vi "Perform Measurement.vi"(7 "error in":errorcluster, 8 "Measure Call Context in":refnum<class "Measure Call Context.lvclass">, 10 "measurement configuration":T2={"Mode of operation"=enum."Power on the DUT", "Source resource names"=[], "Load resource names"=[], "Power ON output function"=1006, "Power ON/Source system configuration"=enum."Parallel", "Power ON V/I Source start level"=6.0, "Source stop voltage"=14.0, "Source voltage sweep points"=4, "Source voltage level range"=20.0, "Power ON/Source sense"=1009, "Source limit symmetry"=enum."Asymmetric", "Power ON/Source current/voltage limit range"=25.0, "Source current limit low"=-0.6, "Source current limit high"=25.0, "Source transient response"=1038, "Source voltage gain bandwidth"=2000.0, "Source voltage compensation frequency"=3530.0, "Source voltage pole-zero ratio"=2.0, "Load system configuration"=enum."Parallel", "Load device voltage/current rating"=50.0, "Load start current"=1.0, "Load stop current"=50.0, "Load current sweep points/points per decade"=10, "Load sweep type"="Logarithmic", "Load current level range"=80.0, "Load sense"=1009, "Load limit symmetry"=enum."Symmetric", "Load voltage limit range"=6.0, "Load voltage limit low"=0.0, "Load voltage limit high"=inf, "Load transient response"=1038, "Load current gain bandwidth"=14000.0, "Load current compensation frequency"=180000.0, "Load current pole-zero ratio"=0.3, "DUT setup time"=1.0, "Source delay"=0.005, "Aperture time"=0.005, "Nominal output voltage"=1.0, "Measurement timeout"=10.0} {"Power ON output function" items=["Series", "Parallel", "Manual"]; "Nominal output voltage" format="%#_6pA"; "Source stop voltage" format="%#_6p"; "Load stop current" format="%#_6p"; "Source voltage sweep points" format="%#_6p"; "Load sense" items=["Symmetric", "Asymmetric"]; "Load transient response" items=["Slow"=1041, "Normal"=1038, "Fast"=1039, "Custom"=1042]; "Power ON/Source sense" items=["Symmetric", "Asymmetric"]; "Source transient response" items=["Slow"=1041, "Normal"=1038, "Fast"=1039, "Custom"=1042]; "Load voltage limit high" format="%#_6p"; "Load voltage limit range" format="%#_6p"; "Load current level range" format="%#_6p"; "Source current limit high" format="%#_6p"; "Source current limit low" format="%#_6p"; "Power ON/Source current/voltage limit range" format="%#_6p"; "Source voltage level range" format="%#_6p"}) -> (0 "error out":errorcluster, 1 "Measure Call Context out":refnum<class "Measure Call Context.lvclass">, 3 "measurement results":T1)   [LabVIEW 2021, in "Eff And Load Reg_Channel Ganging.lvlib"]
doc: "Perform the calling of API in proper sequence to take Efficency and Load regulation measurement in different configurations of source and load like\n\nSingle-Single\nSingle-Ganged\nGanged-Single\nGanged-Ganged"
uses:
  Eff And Load Reg_Channel Ganging.lvlib
  shared subVIs/ctl/NIDCPower_channel_ganging - ctl - ganged config.ctl
  shared subVIs/ctl/NIDCPower_channel_ganging - ctl - channel mode.ctl
  shared/Single/controls/Initialize Resource Config-Single.ctl
  shared/Ganging/controls/Initialize Resource Config-Ganging.ctl
  shared subVIs/ctl/NIDCPower_channel_ganging - ctl - ganged session.ctl
  <instrlib>/niDCPower/nidcpower.llb/niDCPower Wait For Event - Event.ctl
  shared/Single/controls/Source to Sequence Config-Single.ctl
  shared/Ganging/controls/Source to Sequence Config-Ganging.ctl
  shared/Single/controls/Load to Sequence Config-Single.ctl
  shared/Ganging/controls/Load to Sequence Config-Ganging.ctl
  shared/Common/controls/Start and Wait for Event.ctl
  shared/Ganging/controls/Abort Single Point-Ganging.ctl
  shared/Single/controls/Abort Single Point-Single.ctl
  <instrlib>/niDCPower/nidcpower.llb/niDCPower Output Function.ctl
  Measurement Results.ctl
  Controls/Efficency perform meaasurement.ctl
  Controls/Efficency fetch measurement control.ctl
  <vilib>/Plug-In SDKs/Measurements/Measure Call Context/Measure Call Context.lvclass
  Measurement Configuration.ctl
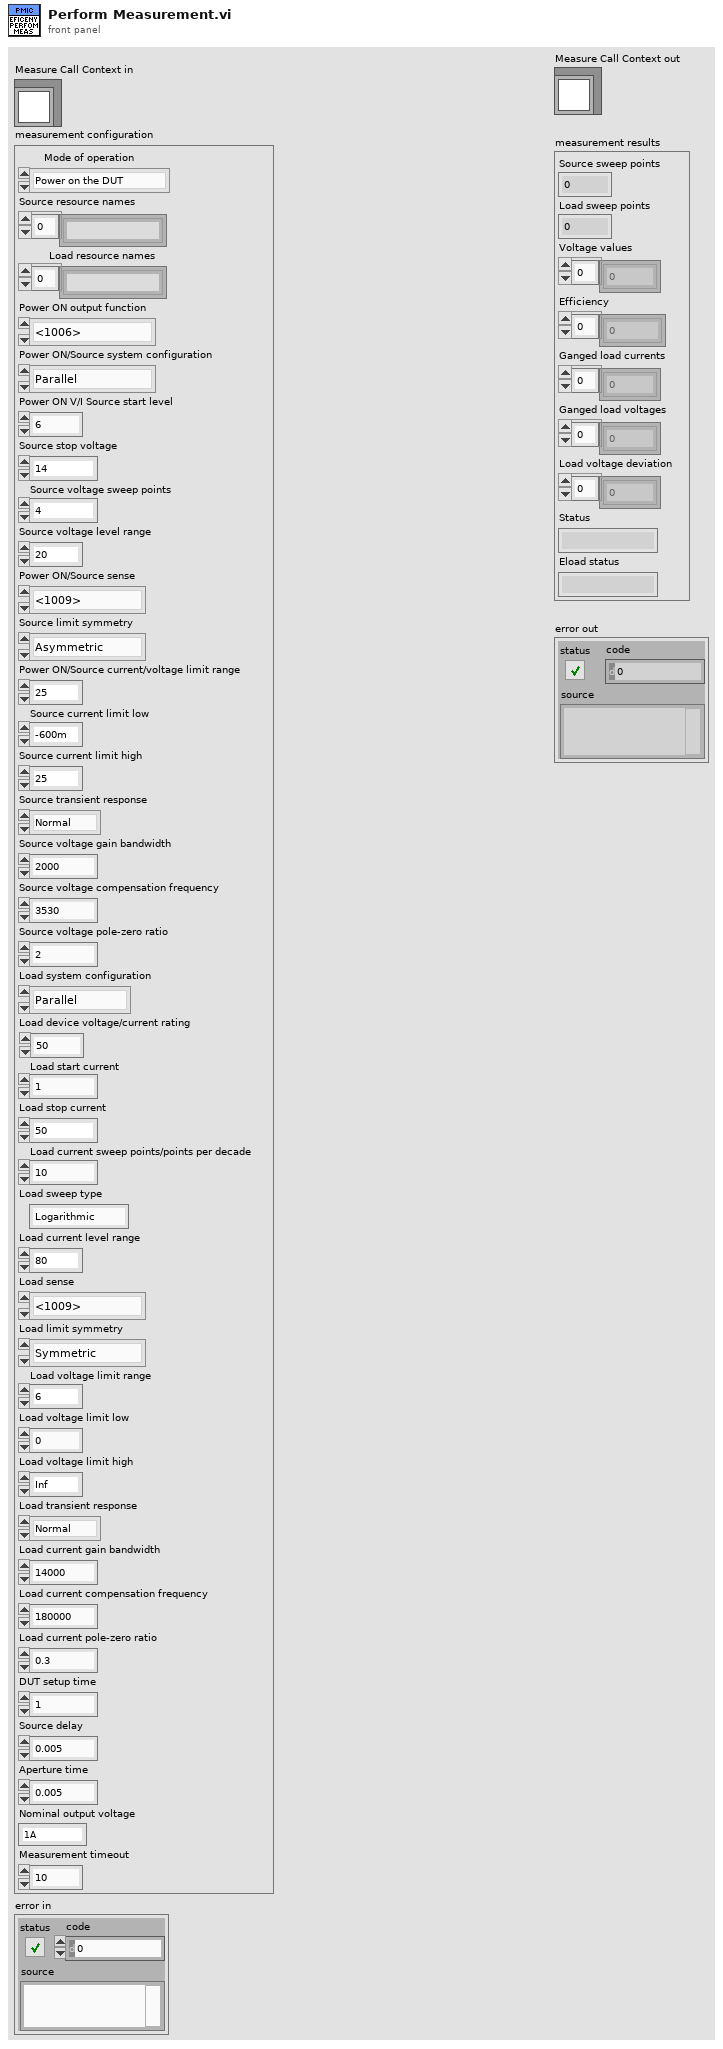
[diagram p1: front panel]
types:
  T1 = typedef "Eff And Load Reg_Channel Ganging.lvlib/Measurement Results.ctl" = cluster{"Source sweep points":i32, "Load sweep points":i32, "Voltage values":dbl[], "Efficiency":dbl[], "Ganged load currents":dbl[], "Ganged load voltages":dbl[], "Load voltage deviation":dbl[], "Status":string, "Eload status":string}
  T2 = typedef "Eff And Load Reg_Channel Ganging.lvlib/Measurement Configuration.ctl" = cluster{"Mode of operation":enum32{"Power on the DUT", "Perform measurement", "Power off the DUT"}, "Source resource names":string[], "Load resource names":string[], "Power ON output function":i32, "Power ON/Source system configuration":enum32{"Series", "Parallel", "Manual"}, "Power ON V/I Source start level":dbl, "Source stop voltage":dbl, "Source voltage sweep points":i32, "Source voltage level range":dbl, "Power ON/Source sense":i32, "Source limit symmetry":enum32{"Symmetric", "Asymmetric"}, "Power ON/Source current/voltage limit range":dbl, "Source current limit low":dbl, "Source current limit high":dbl, "Source transient response":i32, "Source voltage gain bandwidth":dbl, "Source voltage compensation frequency":dbl, "Source voltage pole-zero ratio":dbl, "Load system configuration":enum32{"Series", "Parallel", "Manual"}, "Load device voltage/current rating":dbl, "Load start current":dbl, "Load stop current":dbl, "Load current sweep points/points per decade":i32, "Load sweep type":string, "Load current level range":dbl, "Load sense":i32, "Load limit symmetry":enum32{"Symmetric", "Asymmetric"}, "Load voltage limit range":dbl, "Load voltage limit low":dbl, "Load voltage limit high":dbl, "Load transient response":i32, "Load current gain bandwidth":dbl, "Load current compensation frequency":dbl, "Load current pole-zero ratio":dbl, "DUT setup time":dbl, "Source delay":dbl, "Aperture time":dbl, "Nominal output voltage":dbl, "Measurement timeout":dbl}
  T3 = typedef "Eff And Load Reg_Channel Ganging.lvlib/Efficency perform meaasurement.ctl" = cluster{"Source Ganged Session Out":T4, "Load Ganged Session Out":T4, "Source sweep values":dbl[], "Source sweep points":i32, "Load sweep values":dbl[], "Load sweep points":i32, "Source Master/Single resource name":string, "Source Slave resource name":string[], "Load Master/Single resource name":string, "Load Slave resource name":string[], "Load ganged/single":bool, "Source ganged/single":bool, "Source trigger":string, "measure trigger":string, "Source channel name":string, "Load channel name":string, "Source session out":refnum<k15>, "Load session out":refnum<k15>, "measurement results":T1, "Number of Eload used":i32}
  T4 = typedef "NIDCPower_channel_ganging - ctl - ganged session.ctl" = cluster{"Ganged Config":T5, "Session List":refnum<k15>[], "Session Mode":T6[], "Channel":string[]}
  T5 = typedef "NIDCPower_channel_ganging - ctl - ganged config.ctl" = enum32{"Series", "Parallel", "Manual"}
  T6 = typedef "NIDCPower_channel_ganging - ctl - channel mode.ctl" = enum32{"Master", "Slave", "Slave - Inverted"}
  T7 = typedef "Initialize Resource Config-Single.ctl" = cluster{"Resource name":string, "Voltage/current level":dbl, "Voltage/current level range":dbl, "Voltage/current limit range":dbl, "Voltage/current limit low":dbl, "Voltage/current limit high":dbl, "Output function":i32, "Sense":i32, "Transient response":i32, "Voltage/current gain bandwidth":dbl, "Voltage/current compensation frequency":dbl, "Voltage/current pole-zero ratio":dbl, "DUT set-up time":dbl, "Limit symmetry":enum32{"Symmetric", "Asymmetric"}}
  T8 = typedef "Initialize Resource Config-Ganging.ctl" = cluster{"Master resource name ":string, "Slave resource names":string[], "System configuration":enum32{"Series", "Parallel", "Manual"}, "Voltage/current level":dbl, "Voltage/current level range":dbl, "Limit symmetry":enum32{"Symmetric", "Asymmetric"}, "Voltage/current limit range":dbl, "Voltage/current limit low":dbl, "Voltage/current limit high":dbl, "Output function":i32, "Sense":i32, "Transient response":i32, "Voltage/current gain bandwith":dbl, "Voltage/current compensation frequency":dbl, "Voltage/current pole-zero ratio":dbl, "DUT set-up time":dbl}
  T9 = typedef "Source to Sequence Config-Single.ctl" = cluster{"Source channel name":string, "Source out":refnum<k15>, "Source sweep values":dbl[], "Load sweep points":i32, "Source output function":i32, "Source transient response":i32, "Source voltage/current gain bandwidth":dbl, "Source voltage/current compensation frequency":dbl, "Source voltage/current pole-zero ratio":dbl, "Source aperture time":dbl, "Source source delay":dbl}
  T10 = typedef "Source to Sequence Config-Ganging.ctl" = cluster{"Source Ganged Session Out":cluster{"Ganged Config":T5, "Session List":refnum<k15>[], "Session Mode":T6[], "Channel":string[]}, "Source sweep values":dbl[], "Load sweep points":i32, "Source output function":i32, "Source transient response":i32, "Source voltage/current gain bandwidth":dbl, "Source voltage/current compensation frequency":dbl, "Source voltage/current pole-zero ratio":dbl, "Source aperture time":dbl, "Source source delay":dbl}
  T11 = typedef "Load to Sequence Config-Single.ctl" = cluster{"Load channel name":string, "Load out":refnum<k15>, "Load sweep values":dbl[], "Source sweep points":i32, "Load output function":i32, "Load transient response":i32, "Load voltage/current gain bandwidth":dbl, "Load voltage/current compensation frequency":dbl, "Load voltage/current pole-zero ratio":dbl, "Load aperture time":dbl, "Load source delay":dbl, "Load measure trigger":string, "Load source trigger":string}
  T12 = typedef "Load to Sequence Config-Ganging.ctl" = cluster{"Load Ganged Session Out":cluster{"Ganged Config":T5, "Session List":refnum<k15>[], "Session Mode":T6[], "Channel":string[]}, "Load sweep values":dbl[], "Source sweep points":i32, "Load output function":i32, "Load transient response":i32, "Load voltage/current gain bandwidth":dbl, "Load voltage/current compensation frequency":dbl, "Load voltage/current pole-zero ratio":dbl, "Load aperture time":dbl, "Load source delay":dbl, "Load measure trigger":string, "Load source trigger":string}
  T13 = enum16{"SOURCE AND LOAD OFF", "SOURCE ON", "LOAD ON", "SOURCE AND LOAD ON"}
  T14 = typedef "Start and Wait for Event.ctl" = cluster{"Source Ganged Session Out":T4, "Load Ganged Session Out":T4, "Source session out":refnum<k15>, "Load session out":refnum<k15>, "event":T15, "Source channel name":string, "Load channel name":string, "Load Source ON/OFF":enum16{"SOURCE AND LOAD OFF", "SOURCE ON", "LOAD ON", "SOURCE AND LOAD ON"}, "Load ganged/single":bool, "Source ganged/single":bool}
  T15 = typedef "niDCPower Wait For Event - Event.ctl" = i32
  T16 = typedef "Eff And Load Reg_Channel Ganging.lvlib/Efficency fetch measurement control.ctl" = cluster{"Load,Source ON&OFF":u32, "Source Ganged Session Out":T4, "Load Ganged Session Out":T4, "Source sweep values":dbl[], "Source sweep points":i32, "Load sweep values":dbl[], "Load sweep points":i32, "Load ganged/single":bool, "Source ganged/single":bool, "Source channel name":string, "Load channel name":string, "Source session out":refnum<k15>, "Load session out":refnum<k15>, "measurement results":T1, "Nominal output voltage":dbl, "Measurement timeout":dbl}
  T17 = typedef "Abort Single Point-Ganging.ctl" = cluster{"Ganged Session in":cluster{"Ganged Config":T5, "Session List":refnum<k15>[], "Session Mode":T6[], "Channel":string[]}}
  T18 = typedef "Abort Single Point-Single.ctl" = cluster{"Resource out":refnum<k15>, "Resource channel name":string}
  T19 = enum32{"Power on the DUT", "Perform measurement", "Power off the DUT"}
  T20 = typedef "niDCPower Output Function.ctl" = i32
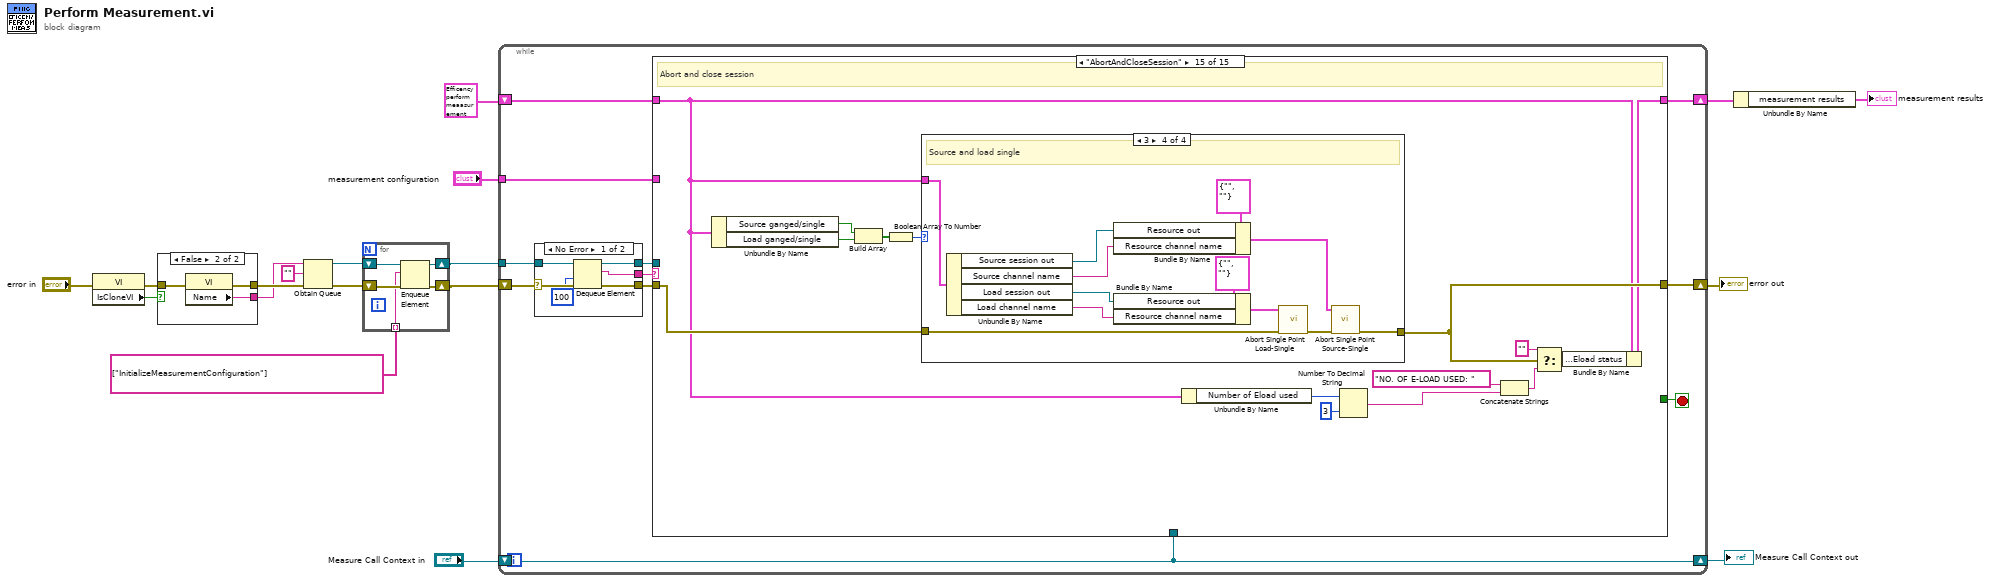
[diagram p0: block diagram]
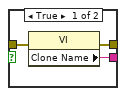
[diagram p2: hidden frame]
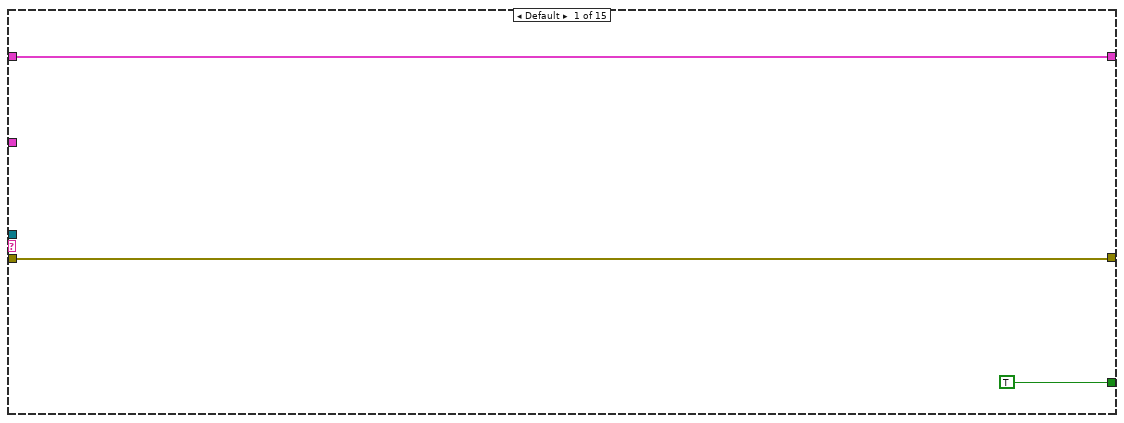
[diagram p3: hidden frame]
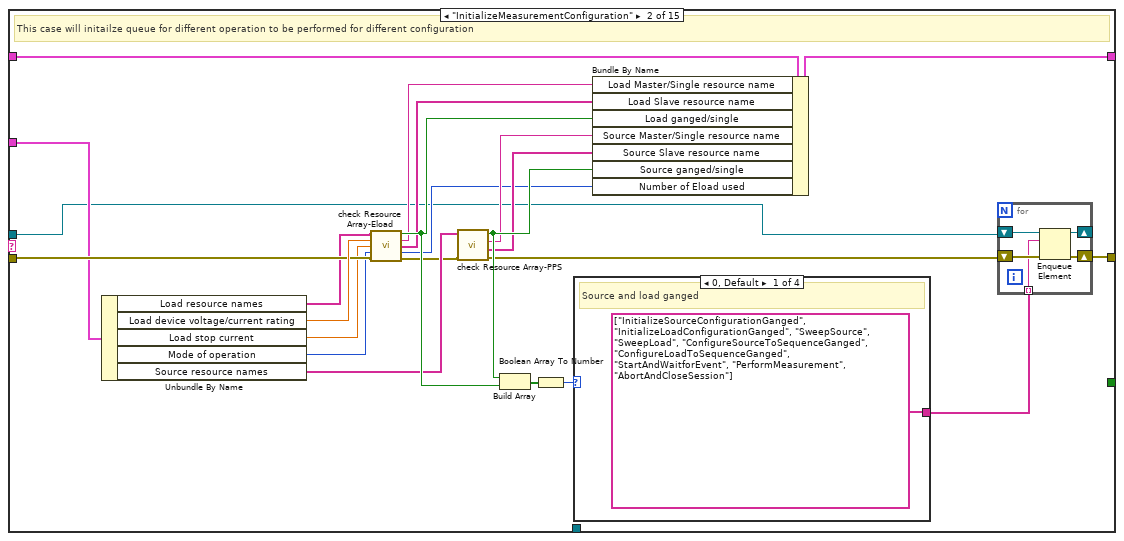
[diagram p4: hidden frame]
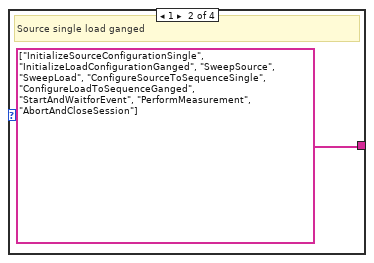
[diagram p5: hidden frame]
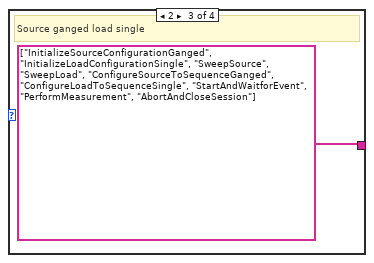
[diagram p6: hidden frame]
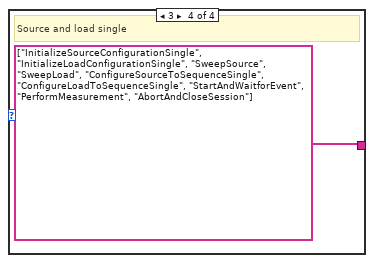
[diagram p7: hidden frame]
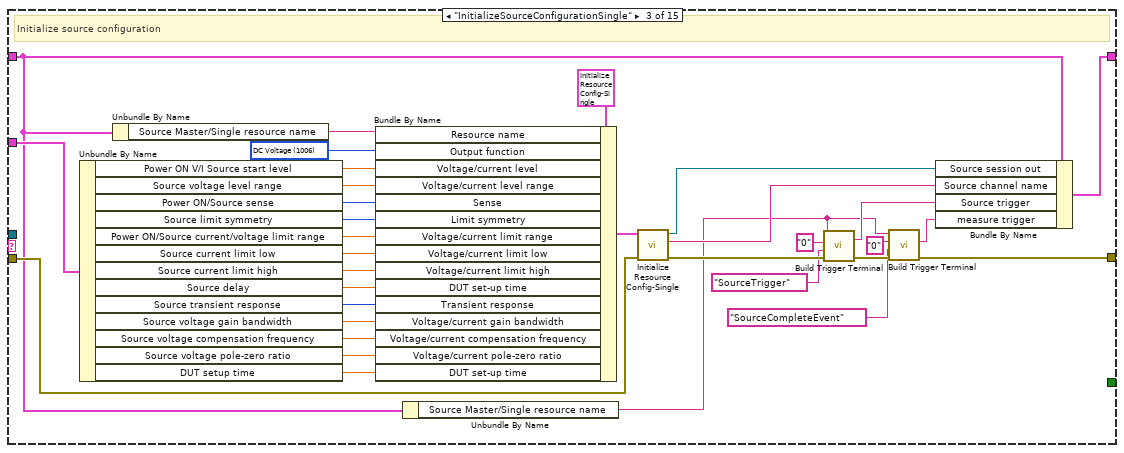
[diagram p8: hidden frame]
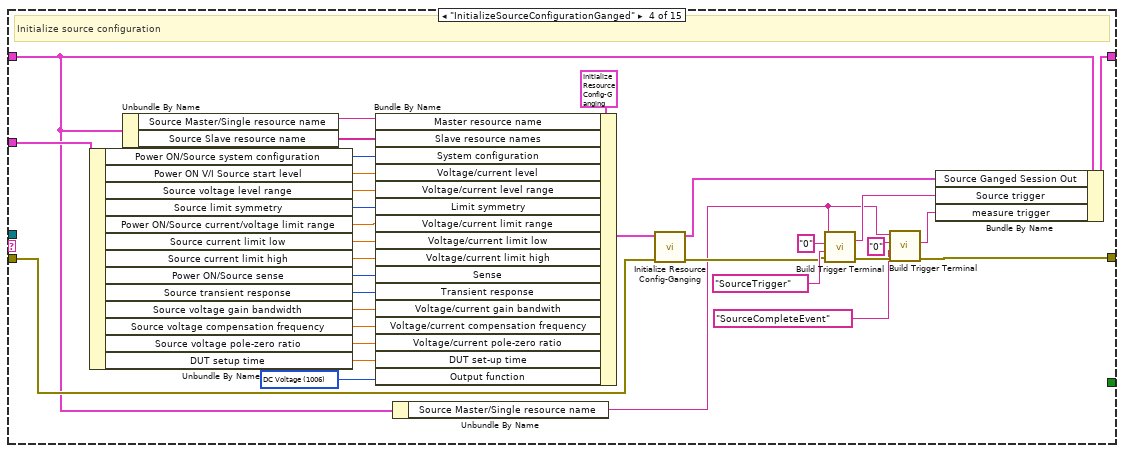
[diagram p9: hidden frame]
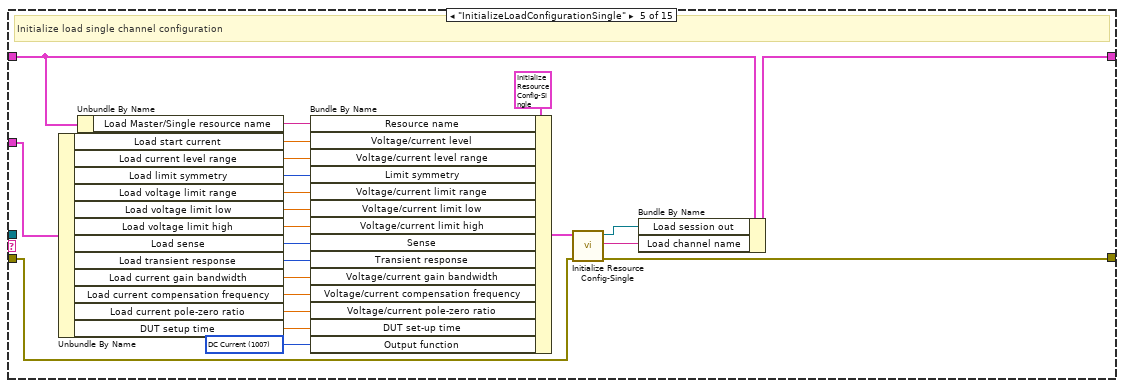
[diagram p10: hidden frame]
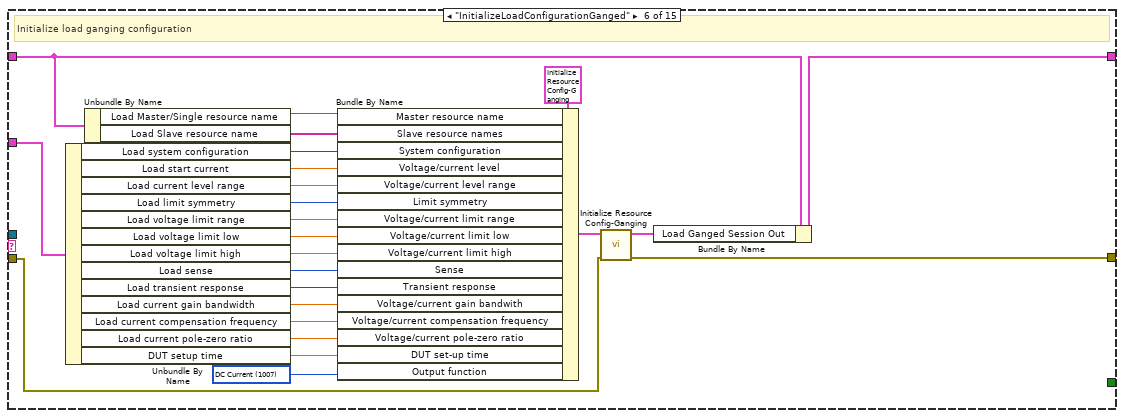
[diagram p11: hidden frame]
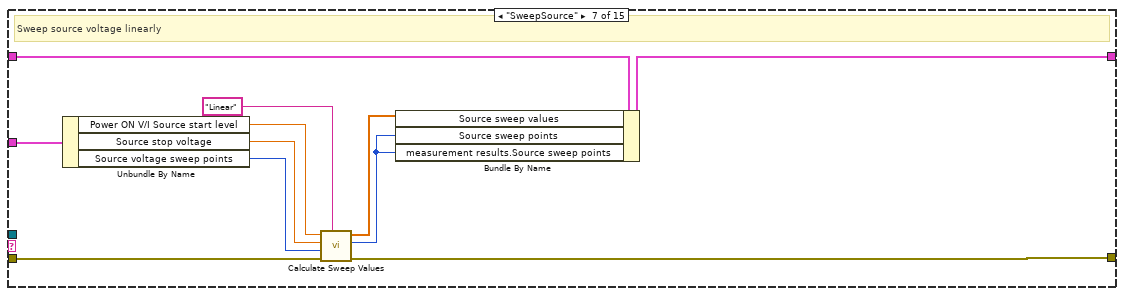
[diagram p12: hidden frame]
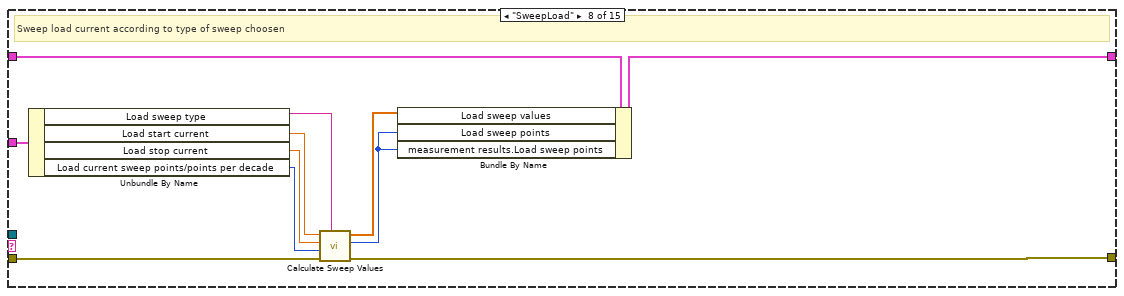
[diagram p13: hidden frame]
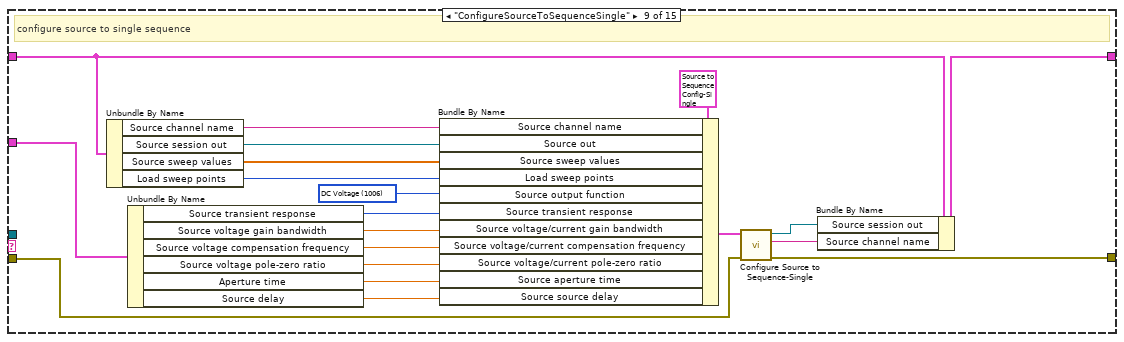
[diagram p14: hidden frame]
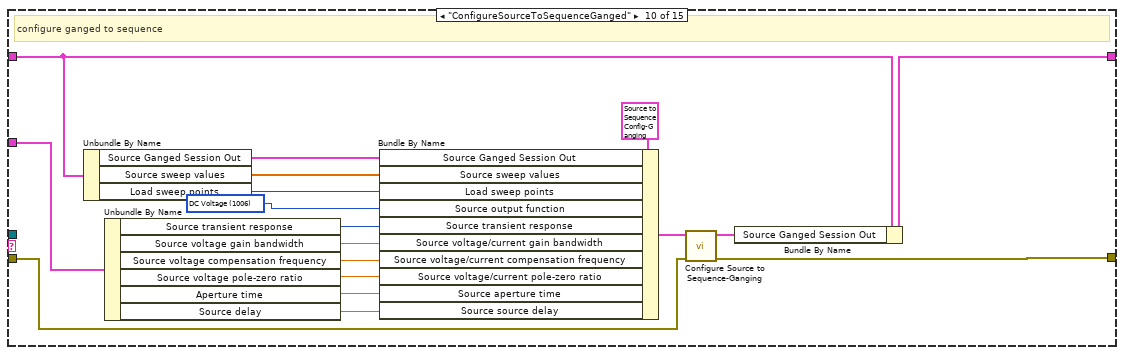
[diagram p15: hidden frame]
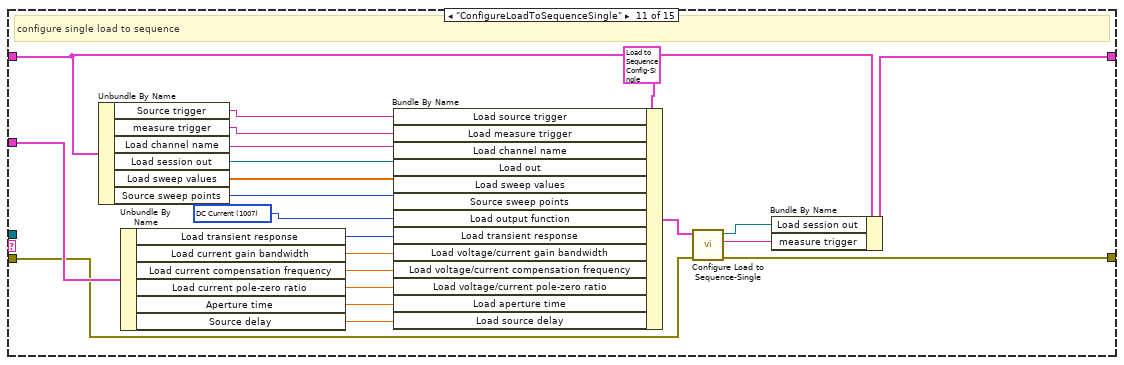
[diagram p16: hidden frame]
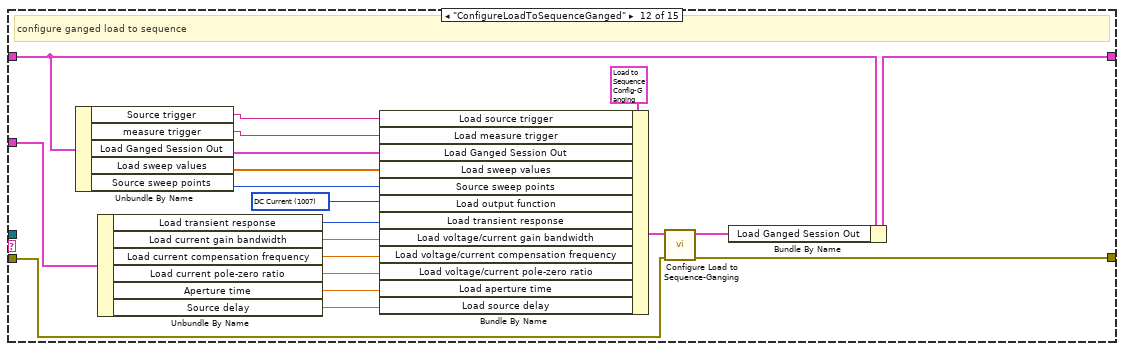
[diagram p17: hidden frame]
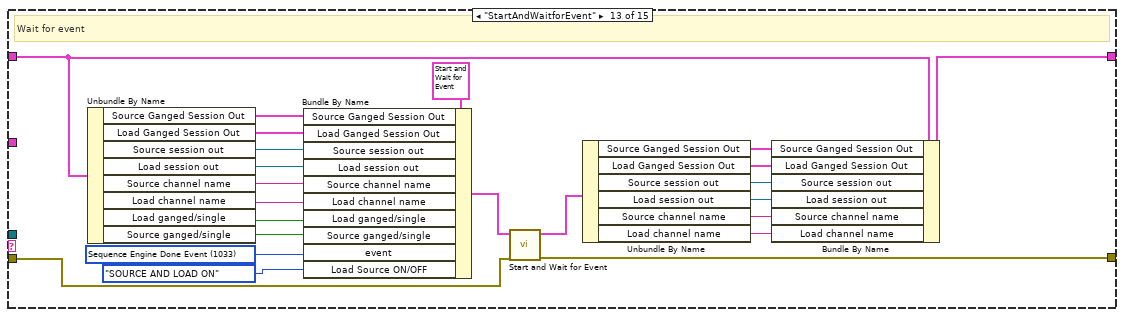
[diagram p18: hidden frame]
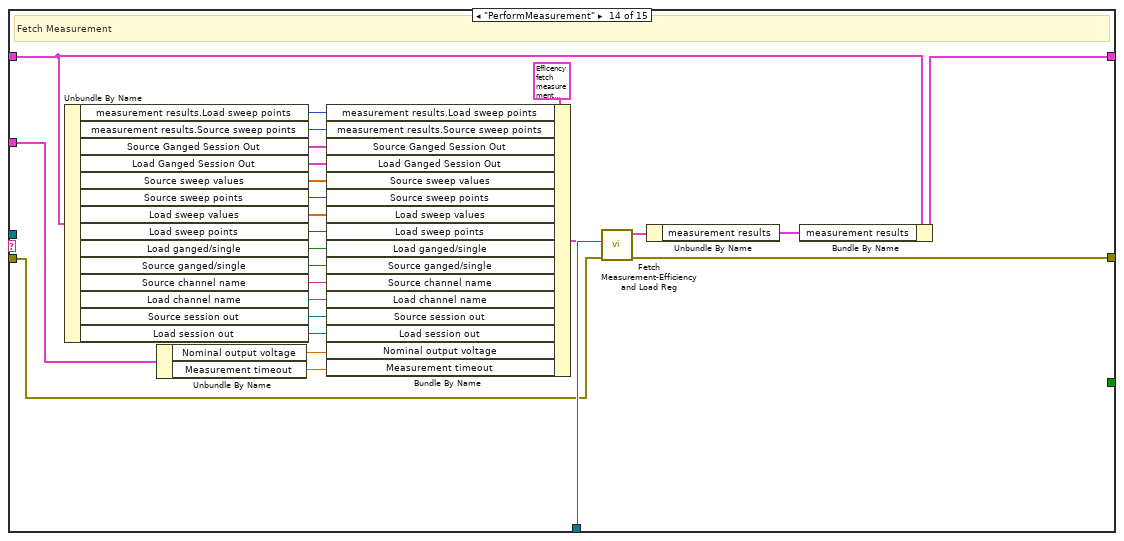
[diagram p19: hidden frame]
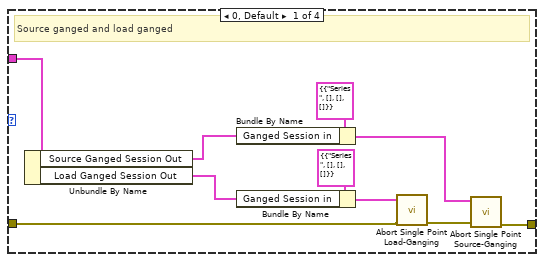
[diagram p20: hidden frame]
diagram:
  n1 = property class="VI"(error in="error in") -> (error out=w13:errorcluster, "IsCloneVI"=w12:bool)  [unwired: 1 in, 1 out]
  n2 = case shown="False" w12 {
    tunnel: [w21 w24] -> w8
    tunnel: [w20 w23] -> w7
    tunnel: w13 -> [w19 w22]
    frame True {
      n3 = property class="VI"(error in=w19) -> (error out=w21:errorcluster, "Clone Name"=w20:string)  [unwired: 1 in, 1 out]
    }
    frame False {
      n4 = property class="VI"(error in=w22) -> (error out=w24:errorcluster, "Name"=w23:string)  [unwired: 1 in, 1 out]
    }
  }
  n5 = Obtain Queue(name (unnamed)=w7, element data type="", error in (no error)=w8) -> (queue out=w10:refnum<queue>, error out=w11:errorcluster)  [unwired: 2 in, 1 out]
  n6 = for {
    shift-right: [w28] -> w5
    shift-left: w10 -> [w26]
    shift-right: [w27] -> w4
    shift-left: w11 -> [w29]
    tunnel: string[] ["InitializeMeasurementConfiguration"] ("Step sequence") -> [w25] mode=indexing
    n7 = Enqueue Element(queue=w26, element=w25, error in (no error)=w29) -> (queue out=w28:refnum<queue>, error out=w27:errorcluster)  [unwired: 1 in, 1 out]
  }
  n8 = while {
    tunnel: w5 -> [w40]
    shift-right: [w34] -> w15
    shift-left: T3 {"Source Ganged Session Out"={"Ganged Config"=enum."Series", "Session List"=[], "Session Mode"=[], "Channel"=[]}, "Load Ganged Session Out"={"Ganged Config"=enum."Series", "Session List"=[], "Session Mode"=[], "Channel"=[]}, "Source sweep values"=[], "Source sweep points"=0, "Load sweep values"=[], "Load sweep points"=0, "Source Master/Single resource name"="", "Source Slave resource name"=[], "Load Master/Single resource name"="", "Load Slave resource name"=[], "Load ganged/single"=FALSE, "Source ganged/single"=FALSE, "Source trigger"="", "measure trigger"="", "Source channel name"="", "Load channel name"="", "Source session out"="", "Load session out"="", "measurement results"={"Source sweep points"=0, "Load sweep points"=0, "Voltage values"=[], "Efficiency"=[], "Ganged load currents"=[], "Ganged load voltages"=[], "Load voltage deviation"=[], "Status"="", "Eload status"=""}, "Number of Eload used"=0} ("Efficency perform measurement") -> [w35]
    shift-right: [w30] -> w18
    shift-left: w4 -> [w39]
    shift-right: [w33] -> w16
    shift-left: "Measure Call Context in" -> [w33]
    tunnel: "measurement configuration" -> [w31]
    stop <- w32 stop-if-true
    n9 = case shown="No Error" w39 {
      selector: w39 -> [w403 w407]
      tunnel: w40 -> [w405 w406]
      tunnel: [w404 "Exit" ("t")] -> w38
      tunnel: [w402 w407] -> w36
      tunnel: [w400 w406] -> w37
      frame No Error {
        n10 = Dequeue Element(queue=w405, timeout in ms (-1)=100, error in (no error)=w403) -> (queue out=w400:refnum<queue>, element=w404:string, error out=w402:errorcluster)  [unwired: 1 out]
      }
      frame Error {
      }
    }
    n11 = case shown="\"AbortAndCloseSession\"" w38 {
      tunnel: w37 -> [_ w50 _ _ _ _ _ _ _ _ _ _ _ _ _]
      tunnel: w36 -> [w42 w55 w90 w124 w145 w184 w199 w210 w215 w235 w255 w277 w296 w317 w355]
      tunnel: w35 -> [w43 w49 w83 w109 w147 w183 w194 w204 w227 w245 w267 w288 w304 w337 w343]
      tunnel: [w43 w47 w93 w110 w146 w182 w191 w203 w228 w248 w270 w290 w303 w338 w344] -> w34
      tunnel: w33 -> [_ _ _ _ _ _ _ _ _ _ _ _ _ w323 _]
      tunnel: [TRUE _ _ _ _ _ _ _ _ _ _ _ _ _ TRUE] -> w32
      tunnel: w31 -> [_ w54 w108 w125 w162 w185 w198 w209 w226 w246 w266 w287 _ w319 _]
      tunnel: [w42 w48 w84 w111 w144 w167 w190 w201 w214 w234 w254 w276 w295 w339 w345] -> w30
      frame Default {
      }
      frame "InitializeMeasurementConfiguration" {
        # "This case will initailze queue for different operation to be performed for different configuration"
        n12 = Unbundle By Name(w54) -> ("Load resource names"=w44:string[], "Load device voltage/current rating"=w66:dbl, "Load stop current"=w46:dbl, "Mode of operation"=w45:T19, "Source resource names"=w59:string[])
        n13 = call "check Resource Array-Eload.vi"("Resource names"=w44, "Device current rating"=w66, "Expected current level"=w46, "Mode of operation"=w45, "error in"=w55) -> ("Single or ganged configuration"=w64:bool, "Single/Master resouce name"=w60:string, "Slave resource names"=w61:string[], "Number of devices used"=w56:i32, "error out"=w51:errorcluster)  [unwired: 6 in]
        n14 = call "check Resource Array-PPS.vi"("error in"=w51, "Resource names"=w59) -> ("error out"=w57:errorcluster, "Slave resource names"=w63:string[], "Single/Master resouce names"=w62:string, "Single or ganged configuration"=w65:bool)  [unwired: 6 in]
        n15 = Build Array(w65, w64) -> (w53:bool[])
        n16 = Boolean Array To Number(Boolean array=w53) -> (number=w52:u32)
        n17 = case shown="0, Default" w52 {
          tunnel: [string[] ["InitializeSourceConfigurationGanged", "InitializeLoadConfigurationGanged", "SweepSource", "SweepLoad", "ConfigureSourceToSequenceGanged", "ConfigureLoadToSequenceGanged", "StartAndWaitforEvent", "PerformMeasurement", "AbortAndCloseSession"] ("Step sequence") string[] ["InitializeSourceConfigurationSingle", "InitializeLoadConfigurationGanged", "SweepSource", "SweepLoad", "ConfigureSourceToSequenceSingle", "ConfigureLoadToSequenceGanged", "StartAndWaitforEvent", "PerformMeasurement", "AbortAndCloseSession"] ("Step sequence") string[] ["InitializeSourceConfigurationGanged", "InitializeLoadConfigurationSingle", "SweepSource", "SweepLoad", "ConfigureSourceToSequenceGanged", "ConfigureLoadToSequenceSingle", "StartAndWaitforEvent", "PerformMeasurement", "AbortAndCloseSession"] ("Step sequence") string[] ["InitializeSourceConfigurationSingle", "InitializeLoadConfigurationSingle", "SweepSource", "SweepLoad", "ConfigureSourceToSequenceSingle", "ConfigureLoadToSequenceSingle", "StartAndWaitforEvent", "PerformMeasurement", "AbortAndCloseSession"] ("Step sequence")] -> w58
          frame 0, Default {
            # "Source and load ganged"
          }
          frame 1 {
            # "Source single load ganged"
          }
          frame 2 {
            # "Source ganged load single"
          }
          frame 3 {
            # "Source and load single"
          }
        }
        n18 = Bundle By Name(cluster=w49, "Load Master/Single resource name"=w60, "Load Slave resource name"=w61, "Load ganged/single"=w64, "Source Master/Single resource name"=w62, "Source Slave resource name"=w63, "Source ganged/single"=w65, "Number of Eload used"=w56) -> (w47:T3)
        n19 = for {
          shift-right: [w73] -> _
          shift-left: w50 -> [w75]
          shift-right: [w72] -> w48
          shift-left: w57 -> [w74]
          tunnel: w58 -> [w71] mode=indexing
          n20 = Enqueue Element(queue=w75, element=w71, error in (no error)=w74) -> (queue out=w73:refnum<queue>, error out=w72:errorcluster)  [unwired: 1 in, 1 out]
        }
      }
      frame "InitializeSourceConfigurationSingle" {
        w88 = T20 1006 items=["DC Voltage"=1006, "DC Current"=1007, "Pulse Voltage"=1049, "Pulse Current"=1050] ("output function")
        # "Initialize source configuration"
        n21 = Unbundle By Name(w108) -> ("Power ON V/I Source start level"=w107:dbl, "Source voltage level range"=w106:dbl, "Power ON/Source sense"=w105:i32, "Source limit symmetry"=w104:enum32{"Symmetric", "Asymmetric"}, "Power ON/Source current/voltage limit range"=w103:dbl, "Source current limit low"=w102:dbl, "Source current limit high"=w101:dbl, "Source delay"=w89:dbl, "Source transient response"=w100:i32, "Source voltage gain bandwidth"=w99:dbl, "Source voltage compensation frequency"=w98:dbl, "Source voltage pole-zero ratio"=w97:dbl, "DUT setup time"=w87:dbl)
        n22 = Unbundle By Name(w83) -> ("Source Master/Single resource name"=w94:string)
        n23 = Bundle By Name(cluster=T7 {"Resource name"="", "Voltage/current level"=0.0, "Voltage/current level range"=0.0, "Voltage/current limit range"=0.0, "Voltage/current limit low"=0.0, "Voltage/current limit high"=inf, "Output function"=1007, "Sense"=1009, "Transient response"=1038, "Voltage/current gain bandwidth"=0.0, "Voltage/current compensation frequency"=0.0, "Voltage/current pole-zero ratio"=0.0, "DUT set-up time"=0.0, "Limit symmetry"=enum."Symmetric"} ("Initialize Resource Config - Single"), "Resource name"=w94, "Output function"=w88, "Voltage/current level"=w107, "Voltage/current level range"=w106, "Sense"=w105, "Limit symmetry"=w104, "Voltage/current limit range"=w103, "Voltage/current limit low"=w102, "Voltage/current limit high"=w101, "DUT set-up time"=w89, "Transient response"=w100, "Voltage/current gain bandwidth"=w99, "Voltage/current compensation frequency"=w98, "Voltage/current pole-zero ratio"=w97, "DUT set-up time"=w87) -> (w95:T7)
        n24 = Unbundle By Name(w83) -> ("Source Master/Single resource name"=w76:string)
        n25 = call "Initialize Resource Config-Single.vi"("error in"=w90, "Initialize resource Config - Single"=w95) -> ("error out"=w86:errorcluster, "channel name"=w92:string, "instrument handle out"=w91:refnum<k15>)  [unwired: 7 in]
        n26 = call "Build Trigger Terminal.vi"("error in (no error)"=w86, "Trigger/Event Name"="SourceTrigger", "Channel Name"="0", "Resource Name"=w76) -> ("error out"=w85:errorcluster, "Terminal Name"=w78:string)  [unwired: 6 in]
        n27 = call "Build Trigger Terminal.vi"("error in (no error)"=w85, "Trigger/Event Name"="SourceCompleteEvent", "Channel Name"="0", "Resource Name"=w76) -> ("error out"=w84:errorcluster, "Terminal Name"=w79:string)  [unwired: 6 in]
        n28 = Bundle By Name(cluster=w83, "Source session out"=w91, "Source channel name"=w92, "Source trigger"=w78, "measure trigger"=w79) -> (w93:T3)
      }
      frame "InitializeSourceConfigurationGanged" {
        w123 = T20 1006 items=["DC Voltage"=1006, "DC Current"=1007, "Pulse Voltage"=1049, "Pulse Current"=1050] ("output function")
        # "Initialize source configuration"
        n29 = Unbundle By Name(w125) -> ("Power ON/Source system configuration"=w137:enum32{"Series", "Parallel", "Manual"}, "Power ON V/I Source start level"=w136:dbl, "Source voltage level range"=w135:dbl, "Source limit symmetry"=w134:enum32{"Symmetric", "Asymmetric"}, "Power ON/Source current/voltage limit range"=w126:dbl, "Source current limit low"=w127:dbl, "Source current limit high"=w128:dbl, "Power ON/Source sense"=w129:i32, "Source transient response"=w130:i32, "Source voltage gain bandwidth"=w133:dbl, "Source voltage compensation frequency"=w132:dbl, "Source voltage pole-zero ratio"=w131:dbl, "DUT setup time"=w122:dbl)
        n30 = Unbundle By Name(w109) -> ("Source Master/Single resource name"=w139:string, "Source Slave resource name"=w138:string[])
        n31 = Bundle By Name(cluster=T8 {"Master resource name "="", "Slave resource names"=[], "System configuration"=enum."Parallel", "Voltage/current level"=0.0, "Voltage/current level range"=0.0, "Limit symmetry"=enum."Symmetric", "Voltage/current limit range"=0.0, "Voltage/current limit low"=0.0, "Voltage/current limit high"=inf, "Output function"=1007, "Sense"=1009, "Transient response"=1038, "Voltage/current gain bandwith"=0.0, "Voltage/current compensation frequency"=0.0, "Voltage/current pole-zero ratio"=0.0, "DUT set-up time"=0.0} ("Initialize Resource Config - Ganging"), "Master resource name"=w139, "Slave resource names"=w138, "System configuration"=w137, "Voltage/current level"=w136, "Voltage/current level range"=w135, "Limit symmetry"=w134, "Voltage/current limit range"=w126, "Voltage/current limit low"=w127, "Voltage/current limit high"=w128, "Sense"=w129, "Transient response"=w130, "Voltage/current gain bandwith"=w133, "Voltage/current compensation frequency"=w132, "Voltage/current pole-zero ratio"=w131, "DUT set-up time"=w122, "Output function"=w123) -> (w141:T8)
        n32 = Unbundle By Name(w109) -> ("Source Master/Single resource name"=w113:string)
        n33 = call "Initialize Resource Config-Ganging.vi"("error in"=w124, "Initialize Resource Config - Ganging"=w141) -> ("error out"=w114:errorcluster, "Ganged Session Out"=w112:T4)  [unwired: 8 in]
        n34 = call "Build Trigger Terminal.vi"("error in (no error)"=w114, "Trigger/Event Name"="SourceTrigger", "Channel Name"="0", "Resource Name"=w113) -> ("error out"=w121:errorcluster, "Terminal Name"=w116:string)  [unwired: 6 in]
        n35 = call "Build Trigger Terminal.vi"("error in (no error)"=w121, "Trigger/Event Name"="SourceCompleteEvent", "Channel Name"="0", "Resource Name"=w113) -> ("error out"=w111:errorcluster, "Terminal Name"=w117:string)  [unwired: 6 in]
        n36 = Bundle By Name(cluster=w109, "Source Ganged Session Out"=w112, "Source trigger"=w116, "measure trigger"=w117) -> (w110:T3)
      }
      frame "InitializeLoadConfigurationSingle" {
        w143 = T20 1007 items=["DC Voltage"=1006, "DC Current"=1007, "Pulse Voltage"=1049, "Pulse Current"=1050] ("output function")
        # "Initialize load single channel configuration"
        n37 = Unbundle By Name(w162) -> ("Load start current"=w150:dbl, "Load current level range"=w151:dbl, "Load limit symmetry"=w152:enum32{"Symmetric", "Asymmetric"}, "Load voltage limit range"=w153:dbl, "Load voltage limit low"=w154:dbl, "Load voltage limit high"=w155:dbl, "Load sense"=w156:i32, "Load transient response"=w160:i32, "Load current gain bandwidth"=w159:dbl, "Load current compensation frequency"=w158:dbl, "Load current pole-zero ratio"=w157:dbl, "DUT setup time"=w142:dbl)
        n38 = Unbundle By Name(w147) -> ("Load Master/Single resource name"=w161:string)
        n39 = Bundle By Name(cluster=T7 {"Resource name"="", "Voltage/current level"=0.0, "Voltage/current level range"=0.0, "Voltage/current limit range"=0.0, "Voltage/current limit low"=0.0, "Voltage/current limit high"=inf, "Output function"=1007, "Sense"=1009, "Transient response"=1038, "Voltage/current gain bandwidth"=0.0, "Voltage/current compensation frequency"=0.0, "Voltage/current pole-zero ratio"=0.0, "DUT set-up time"=0.0, "Limit symmetry"=enum."Symmetric"} ("Initialize Resource Config - Single"), "Resource name"=w161, "Voltage/current level"=w150, "Voltage/current level range"=w151, "Limit symmetry"=w152, "Voltage/current limit range"=w153, "Voltage/current limit low"=w154, "Voltage/current limit high"=w155, "Sense"=w156, "Transient response"=w160, "Voltage/current gain bandwidth"=w159, "Voltage/current compensation frequency"=w158, "Voltage/current pole-zero ratio"=w157, "DUT set-up time"=w142, "Output function"=w143) -> (w163:T7)
        n40 = call "Initialize Resource Config-Single.vi"("error in"=w145, "Initialize resource Config - Single"=w163) -> ("error out"=w144:errorcluster, "channel name"=w148:string, "instrument handle out"=w149:refnum<k15>)  [unwired: 7 in]
        n41 = Bundle By Name(cluster=w147, "Load session out"=w149, "Load channel name"=w148) -> (w146:T3)
      }
      frame "InitializeLoadConfigurationGanged" {
        w166 = T20 1007 items=["DC Voltage"=1006, "DC Current"=1007, "Pulse Voltage"=1049, "Pulse Current"=1050] ("output function")
        # "Initialize load ganging configuration"
        n42 = Unbundle By Name(w185) -> ("Load system configuration"=w179:enum32{"Series", "Parallel", "Manual"}, "Load start current"=w178:dbl, "Load current level range"=w177:dbl, "Load limit symmetry"=w176:enum32{"Symmetric", "Asymmetric"}, "Load voltage limit range"=w175:dbl, "Load voltage limit low"=w174:dbl, "Load voltage limit high"=w173:dbl, "Load sense"=w172:i32, "Load transient response"=w171:i32, "Load current gain bandwidth"=w170:dbl, "Load current compensation frequency"=w169:dbl, "Load current pole-zero ratio"=w168:dbl, "DUT setup time"=w165:dbl)
        n43 = Unbundle By Name(w183) -> ("Load Master/Single resource name"=w181:string, "Load Slave resource name"=w180:string[])
        n44 = Bundle By Name(cluster=T8 {"Master resource name "="", "Slave resource names"=[], "System configuration"=enum."Parallel", "Voltage/current level"=0.0, "Voltage/current level range"=0.0, "Limit symmetry"=enum."Symmetric", "Voltage/current limit range"=0.0, "Voltage/current limit low"=0.0, "Voltage/current limit high"=inf, "Output function"=1007, "Sense"=1009, "Transient response"=1038, "Voltage/current gain bandwith"=0.0, "Voltage/current compensation frequency"=0.0, "Voltage/current pole-zero ratio"=0.0, "DUT set-up time"=0.0} ("Initialize Resource Config - Ganging"), "Master resource name"=w181, "Slave resource names"=w180, "System configuration"=w179, "Voltage/current level"=w178, "Voltage/current level range"=w177, "Limit symmetry"=w176, "Voltage/current limit range"=w175, "Voltage/current limit low"=w174, "Voltage/current limit high"=w173, "Sense"=w172, "Transient response"=w171, "Voltage/current gain bandwith"=w170, "Voltage/current compensation frequency"=w169, "Voltage/current pole-zero ratio"=w168, "DUT set-up time"=w165, "Output function"=w166) -> (w188:T8)
        n45 = call "Initialize Resource Config-Ganging.vi"("error in"=w184, "Initialize Resource Config - Ganging"=w188) -> ("error out"=w167:errorcluster, "Ganged Session Out"=w187:T4)  [unwired: 8 in]
        n46 = Bundle By Name(cluster=w183, "Load Ganged Session Out"=w187) -> (w182:T3)
      }
      frame "SweepSource" {
        # "Sweep source voltage linearly"
        n47 = Unbundle By Name(w198) -> ("Power ON V/I Source start level"=w197:dbl, "Source stop voltage"=w196:dbl, "Source voltage sweep points"=w195:i32)
        n48 = call "Calculate Sweep Values.vi"("Sweep type"="Linear", "error in"=w199, "Points"=w195, "Stop level"=w196, "Start level"=w197) -> ("error out"=w190:errorcluster, "Sweep points"=w192:i32, "Sweep values"=w193:dbl[])  [unwired: 4 in]
        n49 = Bundle By Name(cluster=w194, "Source sweep values"=w193, "Source sweep points"=w192, "measurement results.Source sweep points"=w192) -> (w191:T3)
      }
      frame "SweepLoad" {
        # "Sweep load current according to type of sweep choosen"
        n50 = Unbundle By Name(w209) -> ("Load sweep type"=w208:string, "Load start current"=w207:dbl, "Load stop current"=w206:dbl, "Load current sweep points/points per decade"=w205:i32)
        n51 = call "Calculate Sweep Values.vi"("Sweep type"=w208, "error in"=w210, "Points"=w205, "Stop level"=w206, "Start level"=w207) -> ("error out"=w201:errorcluster, "Sweep points"=w202:i32, "Sweep values"=w200:dbl[])  [unwired: 4 in]
        n52 = Bundle By Name(cluster=w204, "Load sweep values"=w200, "Load sweep points"=w202, "measurement results.Load sweep points"=w202) -> (w203:T3)
      }
      frame "ConfigureSourceToSequenceSingle" {
        w211 = T20 1006 items=["DC Voltage"=1006, "DC Current"=1007, "Pulse Voltage"=1049, "Pulse Current"=1050] ("output function")
        # "configure source to single sequence"
        n53 = Unbundle By Name(w227) -> ("Source channel name"=w223:string, "Source session out"=w224:refnum<k15>, "Source sweep values"=w225:dbl[], "Load sweep points"=w222:i32)
        n54 = Unbundle By Name(w226) -> ("Source transient response"=w221:i32, "Source voltage gain bandwidth"=w220:dbl, "Source voltage compensation frequency"=w219:dbl, "Source voltage pole-zero ratio"=w218:dbl, "Aperture time"=w217:dbl, "Source delay"=w216:dbl)
        n55 = Bundle By Name(cluster=T9 {"Source channel name"="", "Source out"="", "Source sweep values"=[], "Load sweep points"=0, "Source output function"=1006, "Source transient response"=1038, "Source voltage/current gain bandwidth"=0.0, "Source voltage/current compensation frequency"=0.0, "Source voltage/current pole-zero ratio"=0.0, "Source aperture time"=0.0, "Source source delay"=0.0} ("Source to seq config - Single"), "Source channel name"=w223, "Source out"=w224, "Source sweep values"=w225, "Load sweep points"=w222, "Source output function"=w211, "Source transient response"=w221, "Source voltage/current gain bandwidth"=w220, "Source voltage/current compensation frequency"=w219, "Source voltage/current pole-zero ratio"=w218, "Source aperture time"=w217, "Source source delay"=w216) -> (w212:T9)
        n56 = call "Configure Source to Sequence-Single.vi"("error in"=w215, "Source to seq config - Single"=w212) -> ("error out"=w214:errorcluster, "Source channel name"=w229:string, "instrument handle out"=w230:refnum<k15>)  [unwired: 7 in]
        n57 = Bundle By Name(cluster=w227, "Source session out"=w230, "Source channel name"=w229) -> (w228:T3)
      }
      frame "ConfigureSourceToSequenceGanged" {
        w231 = T20 1006 items=["DC Voltage"=1006, "DC Current"=1007, "Pulse Voltage"=1049, "Pulse Current"=1050] ("output function")
        # "configure ganged to sequence"
        n58 = Unbundle By Name(w245) -> ("Source Ganged Session Out"=w238:T4, "Source sweep values"=w237:dbl[], "Load sweep points"=w236:i32)
        n59 = Unbundle By Name(w246) -> ("Source transient response"=w239:i32, "Source voltage gain bandwidth"=w240:dbl, "Source voltage compensation frequency"=w241:dbl, "Source voltage pole-zero ratio"=w242:dbl, "Aperture time"=w243:dbl, "Source delay"=w244:dbl)
        n60 = Bundle By Name(cluster=T10 {"Source Ganged Session Out"={"Ganged Config"=enum."Series", "Session List"=[], "Session Mode"=[], "Channel"=[]}, "Source sweep values"=[], "Load sweep points"=0, "Source output function"=1006, "Source transient response"=1038, "Source voltage/current gain bandwidth"=0.0, "Source voltage/current compensation frequency"=0.0, "Source voltage/current pole-zero ratio"=0.0, "Source aperture time"=0.0, "Source source delay"=0.0} ("Source to seq config - Ganging"), "Source Ganged Session Out"=w238, "Source sweep values"=w237, "Load sweep points"=w236, "Source output function"=w231, "Source transient response"=w239, "Source voltage/current gain bandwidth"=w240, "Source voltage/current compensation frequency"=w241, "Source voltage/current pole-zero ratio"=w242, "Source aperture time"=w243, "Source source delay"=w244) -> (w232:T10)
        n61 = call "Configure Source to Sequence-Ganging.vi"("error in"=w235, "Source to seq config - Ganging"=w232) -> ("error out"=w234:errorcluster, "Ganged Session Out"=w247:T4)  [unwired: 8 in]
        n62 = Bundle By Name(cluster=w245, "Source Ganged Session Out"=w247) -> (w248:T3)
      }
      frame "ConfigureLoadToSequenceSingle" {
        w251 = T20 1007 items=["DC Voltage"=1006, "DC Current"=1007, "Pulse Voltage"=1049, "Pulse Current"=1050] ("output function")
        # "configure single load to sequence"
        n63 = Unbundle By Name(w267) -> ("Source trigger"=w249:string, "measure trigger"=w250:string, "Load channel name"=w265:string, "Load session out"=w264:refnum<k15>, "Load sweep values"=w263:dbl[], "Source sweep points"=w262:i32)
        n64 = Unbundle By Name(w266) -> ("Load transient response"=w261:i32, "Load current gain bandwidth"=w260:dbl, "Load current compensation frequency"=w259:dbl, "Load current pole-zero ratio"=w258:dbl, "Aperture time"=w257:dbl, "Source delay"=w256:dbl)
        n65 = Bundle By Name(cluster=T11 {"Load channel name"="", "Load out"="", "Load sweep values"=[], "Source sweep points"=0, "Load output function"=1007, "Load transient response"=1038, "Load voltage/current gain bandwidth"=0.0, "Load voltage/current compensation frequency"=0.0, "Load voltage/current pole-zero ratio"=0.0, "Load aperture time"=0.0, "Load source delay"=0.0, "Load measure trigger"="", "Load source trigger"=""} ("Load to seq config - Single"), "Load source trigger"=w249, "Load measure trigger"=w250, "Load channel name"=w265, "Load out"=w264, "Load sweep values"=w263, "Source sweep points"=w262, "Load output function"=w251, "Load transient response"=w261, "Load voltage/current gain bandwidth"=w260, "Load voltage/current compensation frequency"=w259, "Load voltage/current pole-zero ratio"=w258, "Load aperture time"=w257, "Load source delay"=w256) -> (w252:T11)
        n66 = call "Configure Load to Sequence-Single.vi"("error in"=w255, "Load to seq config - Single"=w252) -> ("error out"=w254:errorcluster, "Load channel Name"=w268:string, "instrument handle out"=w269:refnum<k15>)  [unwired: 7 in]
        n67 = Bundle By Name(cluster=w267, "Load session out"=w269, "measure trigger"=w268) -> (w270:T3)
      }
      frame "ConfigureLoadToSequenceGanged" {
        w273 = T20 1007 items=["DC Voltage"=1006, "DC Current"=1007, "Pulse Voltage"=1049, "Pulse Current"=1050] ("output function")
        # "configure ganged load to sequence"
        n68 = Unbundle By Name(w288) -> ("Source trigger"=w271:string, "measure trigger"=w272:string, "Load Ganged Session Out"=w286:T4, "Load sweep values"=w285:dbl[], "Source sweep points"=w284:i32)
        n69 = Unbundle By Name(w287) -> ("Load transient response"=w283:i32, "Load current gain bandwidth"=w282:dbl, "Load current compensation frequency"=w281:dbl, "Load current pole-zero ratio"=w280:dbl, "Aperture time"=w279:dbl, "Source delay"=w278:dbl)
        n70 = Bundle By Name(cluster=T12 {"Load Ganged Session Out"={"Ganged Config"=enum."Series", "Session List"=[], "Session Mode"=[], "Channel"=[]}, "Load sweep values"=[], "Source sweep points"=0, "Load output function"=1007, "Load transient response"=1038, "Load voltage/current gain bandwidth"=0.0, "Load voltage/current compensation frequency"=0.0, "Load voltage/current pole-zero ratio"=0.0, "Load aperture time"=0.0, "Load source delay"=0.0, "Load measure trigger"="", "Load source trigger"=""} ("Load to seq config - Ganging"), "Load source trigger"=w271, "Load measure trigger"=w272, "Load Ganged Session Out"=w286, "Load sweep values"=w285, "Source sweep points"=w284, "Load output function"=w273, "Load transient response"=w283, "Load voltage/current gain bandwidth"=w282, "Load voltage/current compensation frequency"=w281, "Load voltage/current pole-zero ratio"=w280, "Load aperture time"=w279, "Load source delay"=w278) -> (w274:T12)
        n71 = call "Configure Load to Sequence-Ganging.vi"("error in"=w277, "Load to seq config - Ganging"=w274) -> ("error out"=w276:errorcluster, "Ganged Session Out"=w289:T4)  [unwired: 8 in]
        n72 = Bundle By Name(cluster=w288, "Load Ganged Session Out"=w289) -> (w290:T3)
      }
      frame "StartAndWaitforEvent" {
        w305 = T15 1033 items=["Source Complete Event"=1030, "Measure Complete Event"=1031, "Sequence Iteration Complete Event"=1032, "Sequence Engine Done Event"=1033, "Pulse Complete Event"=1051, "Ready For Pulse Trigger Event"=1052] ("event")
        # "Wait for event"
        n73 = Unbundle By Name(w304) -> ("Source Ganged Session Out"=w313:T4, "Load Ganged Session Out"=w312:T4, "Source session out"=w311:refnum<k15>, "Load session out"=w310:refnum<k15>, "Source channel name"=w309:string, "Load channel name"=w308:string, "Load ganged/single"=w307:bool, "Source ganged/single"=w306:bool)
        n74 = Bundle By Name(cluster=T14 {"Source Ganged Session Out"={"Ganged Config"=enum."Series", "Session List"=[], "Session Mode"=[], "Channel"=[]}, "Load Ganged Session Out"={"Ganged Config"=enum."Series", "Session List"=[], "Session Mode"=[], "Channel"=[]}, "Source session out"="", "Load session out"="", "event"=1030, "Source channel name"="", "Load channel name"="", "Load Source ON/OFF"=enum."SOURCE AND LOAD OFF", "Load ganged/single"=FALSE, "Source ganged/single"=FALSE} ("Start and wait event config"), "Source Ganged Session Out"=w313, "Load Ganged Session Out"=w312, "Source session out"=w311, "Load session out"=w310, "Source channel name"=w309, "Load channel name"=w308, "Load ganged/single"=w307, "Source ganged/single"=w306, "event"=w305, "Load Source ON/OFF"=T13."SOURCE AND LOAD ON") -> (w292:T14)
        n75 = call "Start and Wait for Event.vi"("error in"=w296, "Start and wait event config"=w292) -> ("error out"=w295:errorcluster, "Start and wait event result"=w294:T14)  [unwired: 7 in]
        n76 = Unbundle By Name(w294) -> ("Source Ganged Session Out"=w302:T4, "Load Ganged Session Out"=w301:T4, "Source session out"=w300:refnum<k15>, "Load session out"=w299:refnum<k15>, "Source channel name"=w298:string, "Load channel name"=w297:string)
        n77 = Bundle By Name(cluster=w304, "Source Ganged Session Out"=w302, "Load Ganged Session Out"=w301, "Source session out"=w300, "Load session out"=w299, "Source channel name"=w298, "Load channel name"=w297) -> (w303:T3)
      }
      frame "PerformMeasurement" {
        # "Fetch Measurement"
        n78 = Unbundle By Name(w337) -> ("measurement results.Load sweep points"=w321:i32, "measurement results.Source sweep points"=w320:i32, "Source Ganged Session Out"=w336:T4, "Load Ganged Session Out"=w335:T4, "Source sweep values"=w334:dbl[], "Source sweep points"=w333:i32, "Load sweep values"=w332:dbl[], "Load sweep points"=w331:i32, "Load ganged/single"=w330:bool, "Source ganged/single"=w329:bool, "Source channel name"=w328:string, "Load channel name"=w327:string, "Source session out"=w326:refnum<k15>, "Load session out"=w325:refnum<k15>)
        n79 = Unbundle By Name(w319) -> ("Nominal output voltage"=w318:dbl, "Measurement timeout"=w314:dbl)
        n80 = Bundle By Name(cluster=T16 {"Load,Source ON&OFF"=0, "Source Ganged Session Out"={"Ganged Config"=enum."Series", "Session List"=[], "Session Mode"=[], "Channel"=[]}, "Load Ganged Session Out"={"Ganged Config"=enum."Series", "Session List"=[], "Session Mode"=[], "Channel"=[]}, "Source sweep values"=[], "Source sweep points"=0, "Load sweep values"=[], "Load sweep points"=0, "Load ganged/single"=FALSE, "Source ganged/single"=FALSE, "Source channel name"="", "Load channel name"="", "Source session out"="", "Load session out"="", "measurement results"={"Source sweep points"=0, "Load sweep points"=0, "Voltage values"=[], "Efficiency"=[], "Ganged load currents"=[], "Ganged load voltages"=[], "Load voltage deviation"=[], "Status"="", "Eload status"=""}, "Nominal output voltage"=0.0, "Measurement timeout"=10.0} ("Efficency fetch measurement"), "measurement results.Load sweep points"=w321, "measurement results.Source sweep points"=w320, "Source Ganged Session Out"=w336, "Load Ganged Session Out"=w335, "Source sweep values"=w334, "Source sweep points"=w333, "Load sweep values"=w332, "Load sweep points"=w331, "Load ganged/single"=w330, "Source ganged/single"=w329, "Source channel name"=w328, "Load channel name"=w327, "Source session out"=w326, "Load session out"=w325, "Nominal output voltage"=w318, "Measurement timeout"=w314) -> (w315:T16)
        n81 = call "Fetch Measurement-Efficiency and Load Reg.vi"("error in"=w317, "Measure Call Context in"=w323, "Efficency fetch measurement"=w315) -> ("error out"=w339:errorcluster, "Efficency fetch measurement"=w324:T16)  [unwired: 7 in]
        n82 = Unbundle By Name(w324) -> ("measurement results"=w322:T1)
        n83 = Bundle By Name(cluster=w337, "measurement results"=w322) -> (w338:T3)
      }
      frame "AbortAndCloseSession" {
        # "Abort and close session"
        n84 = Unbundle By Name(w343) -> ("Source ganged/single"=w352:bool, "Load ganged/single"=w353:bool)
        n85 = Build Array(w352, w353) -> (w351:bool[])
        n86 = Boolean Array To Number(Boolean array=w351) -> (number=w350:u32)
        n87 = case shown="3" w350 {
          tunnel: w343 -> [w365 w376 w387 w397]
          tunnel: [w359 w370 w379 w388] -> w345
          tunnel: w355 -> [w357 w368 w381 w391]
          frame 0, Default {
            # "Source ganged and load ganged"
            n88 = Unbundle By Name(w365) -> ("Source Ganged Session Out"=w363:T4, "Load Ganged Session Out"=w364:T4)
            n89 = Bundle By Name(cluster=T17 {"Ganged Session in"={"Ganged Config"=enum."Series", "Session List"=[], "Session Mode"=[], "Channel"=[]}} ("Ganged Session In"), "Ganged Session in"=w363) -> (w360:T17)
            n90 = Bundle By Name(cluster=T17 {"Ganged Session in"={"Ganged Config"=enum."Series", "Session List"=[], "Session Mode"=[], "Channel"=[]}} ("Ganged Session In"), "Ganged Session in"=w364) -> (w356:T17)
            n91 = call "Abort Single Point Load-Ganging.vi"("error in"=w357, "Ganged Session In"=w356) -> ("error out"=w358:errorcluster)  [unwired: 9 in]
            n92 = call "Abort Single Point Source-Ganging.vi"("error in"=w358, "Ganged Session In"=w360) -> ("error out"=w359:errorcluster)  [unwired: 9 in]
          }
          frame 1 {
            # "Source single load ganged"
            n93 = Unbundle By Name(w376) -> ("Source session out"=w374:refnum<k15>, "Source channel name"=w373:string, "Load Ganged Session Out"=w375:T4)
            n94 = Bundle By Name(cluster=T18 {"Resource out"="", "Resource channel name"=""} ("Abort Single Point - Single"), "Resource out"=w374, "Resource channel name"=w373) -> (w369:T18)
            n95 = Bundle By Name(cluster=T17 {"Ganged Session in"={"Ganged Config"=enum."Series", "Session List"=[], "Session Mode"=[], "Channel"=[]}} ("Ganged Session In"), "Ganged Session in"=w375) -> (w366:T17)
            n96 = call "Abort Single Point Load-Ganging.vi"("error in"=w368, "Ganged Session In"=w366) -> ("error out"=w367:errorcluster)  [unwired: 9 in]
            n97 = call "Abort Single Point Source-Single.vi"("error in"=w367, "Abort Single Point - Single"=w369) -> ("error out"=w370:errorcluster)  [unwired: 9 in]
          }
          frame 2 {
            # "Source ganged load single"
            n98 = Unbundle By Name(w387) -> ("Source Ganged Session Out"=w384:T4, "Load session out"=w386:refnum<k15>, "Load channel name"=w385:string)
            n99 = Bundle By Name(cluster=T18 {"Resource out"="", "Resource channel name"=""} ("Abort Single Point - Single"), "Resource out"=w386, "Resource channel name"=w385) -> (w380:T18)
            n100 = Bundle By Name(cluster=T17 {"Ganged Session in"={"Ganged Config"=enum."Series", "Session List"=[], "Session Mode"=[], "Channel"=[]}} ("Ganged Session In"), "Ganged Session in"=w384) -> (w377:T17)
            n101 = call "Abort Single Point Load-Single.vi"("error in"=w381, "Abort Single Point - Single"=w380) -> ("error out"=w378:errorcluster)  [unwired: 9 in]
            n102 = call "Abort Single Point Source-Ganging.vi"("error in"=w378, "Ganged Session In"=w377) -> ("error out"=w379:errorcluster)  [unwired: 9 in]
          }
          frame 3 {
            # "Source and load single"
            n103 = Unbundle By Name(w397) -> ("Source session out"=w395:refnum<k15>, "Source channel name"=w396:string, "Load session out"=w399:refnum<k15>, "Load channel name"=w398:string)
            n104 = Bundle By Name(cluster=T18 {"Resource out"="", "Resource channel name"=""} ("Abort Single Point - Single"), "Resource out"=w395, "Resource channel name"=w396) -> (w390:T18)
            n105 = Bundle By Name(cluster=T18 {"Resource out"="", "Resource channel name"=""} ("Abort Single Point - Single"), "Resource out"=w399, "Resource channel name"=w398) -> (w392:T18)
            n106 = call "Abort Single Point Load-Single.vi"("error in"=w391, "Abort Single Point - Single"=w392) -> ("error out"=w389:errorcluster)  [unwired: 9 in]
            n107 = call "Abort Single Point Source-Single.vi"("error in"=w389, "Abort Single Point - Single"=w390) -> ("error out"=w388:errorcluster)  [unwired: 9 in]
          }
        }
        n108 = Unbundle By Name(w343) -> ("Number of Eload used"=w342:i32)
        n109 = Number To Decimal String(number=w342, width (-)=i16 3) -> (decimal integer string=w341:string)
        n110 = Concatenate Strings("NO. OF E-LOAD USED: ", w341) -> (w346:string)
        n111 = Select(t="", s=w345, f=w346) -> (s? t:f=w348:string)
        n112 = Bundle By Name(cluster=w343, "measurement results.Eload status"=w348) -> (w344:T3)
      }
    }
  }
  "error out" <- w18
  "Measure Call Context out" <- w16
  n113 = Unbundle By Name(w15) -> ("measurement results"=→"measurement results":T1)
